vi "Adv_GetControlCurrentCapabilities.vi"(8 "error in (no error)":errorcluster, 9 "Setting":T1(ring), 10 "Control":refnum<vi>, 11 "LightField Automation in":refnum<class "LightField Automation.lvclass">) -> (0 "error out":errorcluster, 3 "LightField Automation out":refnum<class "LightField Automation.lvclass">)   [LabVIEW 2013, in "LightField Automation.lvclass"]
uses:
  LightField Automation.lvclass
  C:/Program Files/Princeton Instruments/LightField/PrincetonInstruments.LightFieldAddInSupportServices.dll
  Program Files/Princeton Instruments/LightField/PrincetonInstruments.LightFieldAddInSupportServices.dll
  LightField Automation.lvclass/LightField Automation.ctl
  C:/Program Files/Princeton Instruments/LightField/AddInViews/PrincetonInstruments.LightFieldViewV3.dll
  Program Files/Princeton Instruments/LightField/AddInViews/PrincetonInstruments.LightFieldViewV3.dll
  <vilib>/Utility/error.llb/DialogType.ctl
  TypeDefs/CalibrationLightSource.ctl
  TypeDefs/ADCGain.ctl
  TypeDefs/ADCQuality.ctl
  TypeDefs/CCDCharacteristics.ctl
  TypeDefs/CosmicRayCorrectionMethod.ctl
  TypeDefs/DateFormat.ctl
  TypeDefs/EMIccdGainControlMode.ctl
  TypeDefs/FileFormatLocation.ctl
  TypeDefs/FrameCombinationMethod.ctl
  TypeDefs/IntensifierOptions.ctl
  TypeDefs/IntensifierStatus.ctl
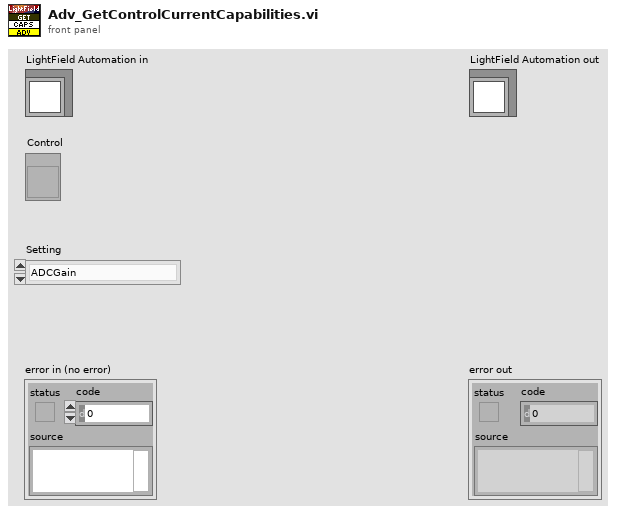
[diagram p1: front panel]
types:
  T1 = enum16{"ADCGain", "ADCQuality", "CalibrationLightSource", "CalibrationMode", "CcdCharacteristics", "CosmicRayCorrectionMethod", "DateFormat", "EMIccdGainControlMode", "FeatureProvider", "FileFormatLocation", "FrameCombinationMethod", "GateTracking", "GatingMode", "GatingSpeed", "IEMGainControlMode", "ImageOrientation", "IntensifierOptions", "IntensifierStatus", "ModulationTracking", "OpticalPortLocation", "OpticalPortShutterType", "OpticalPortType", "OutputSignal", "PhosphorType", "PhotocathodeSensitivity", "PhotonDetectionMode", "PixelDataFormat", "PixelFormat", "ReadoutControlMode", "ReadoutOrientation", "RegionsOfInterestSelection", "SensorTemperatureStatus", "SensorType", "ShutterAccessoryTimingMode", "ShutterTimingMode", "TimeFormat", "TimeStamps", "TriggerCoupling", "TriggerDetermination", "TriggerResponse", "TriggerSource", "TriggerTermination"}
  T2 = typedef "DialogType.ctl" = u16
  T3 = typedef "LVStringsAndValuesArrayTypeDef.ctl" = cluster{"String":string, "Value":ext}[]
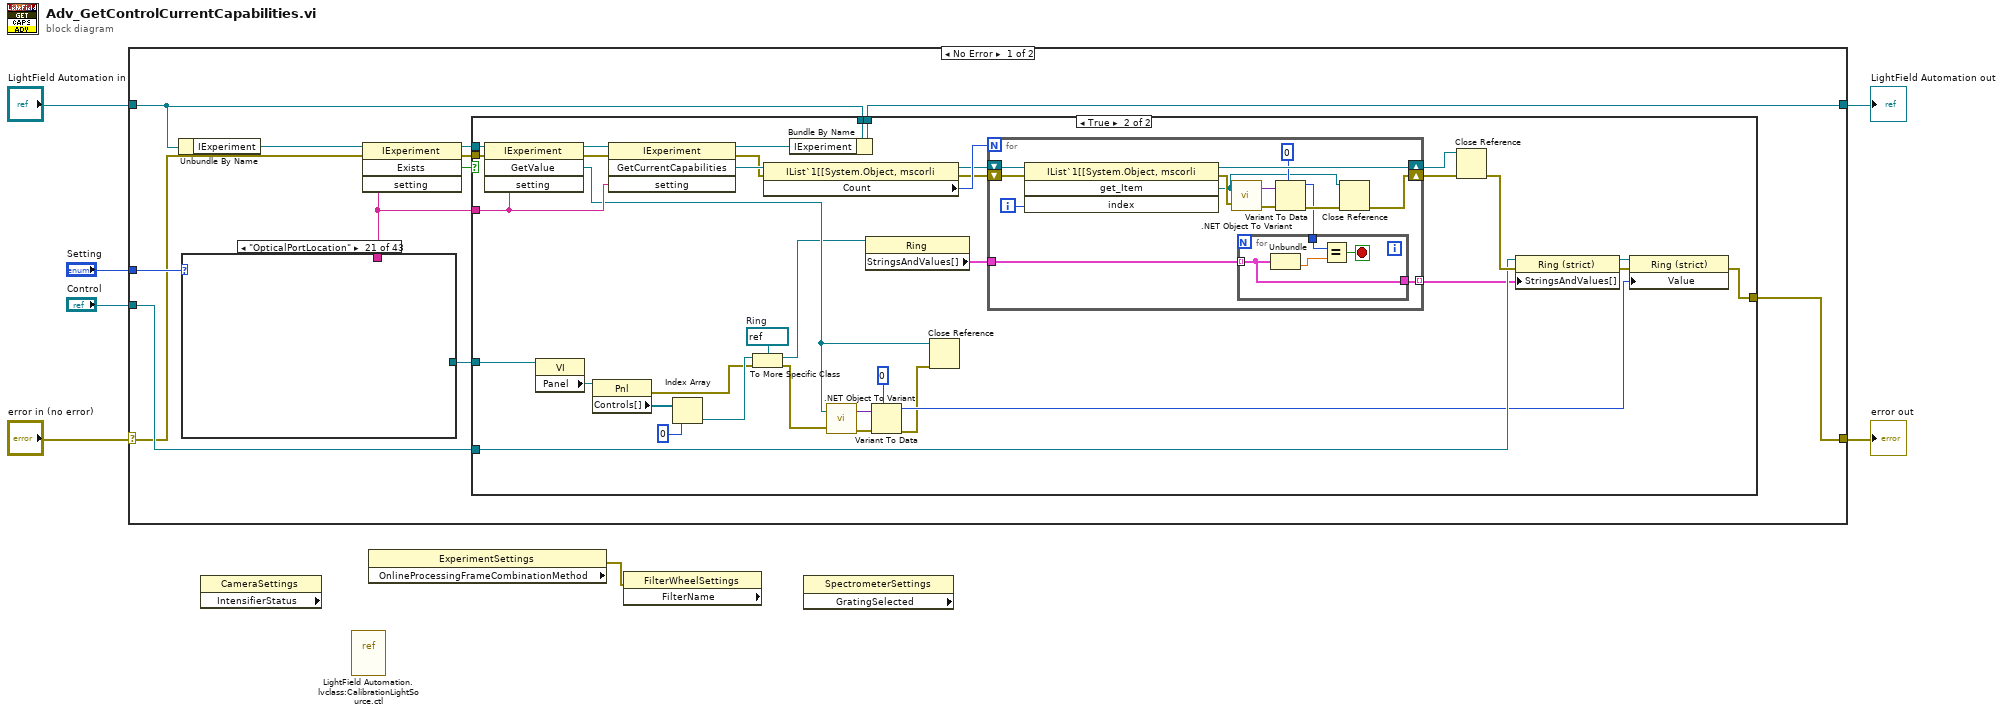
[diagram p0: block diagram]
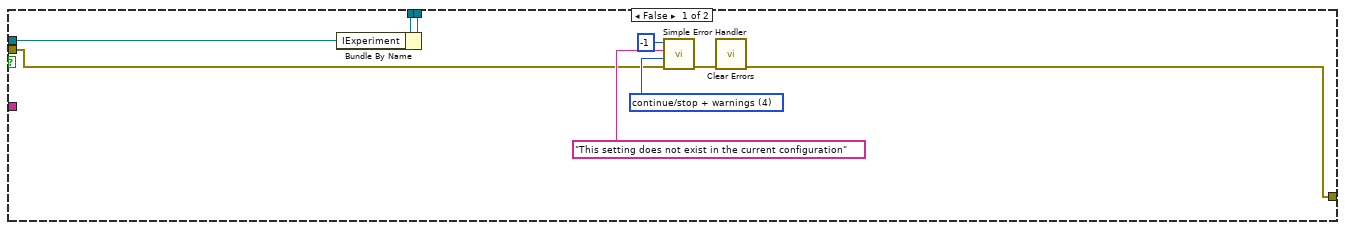
[diagram p2: hidden frame]
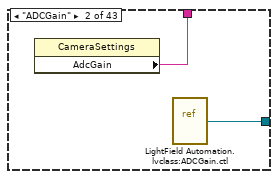
[diagram p4: hidden frame]
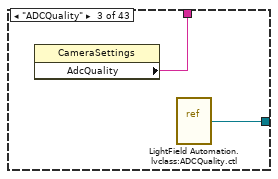
[diagram p5: hidden frame]
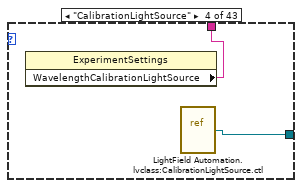
[diagram p6: hidden frame]
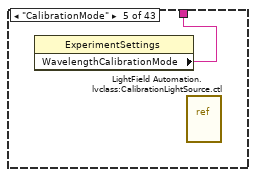
[diagram p7: hidden frame]
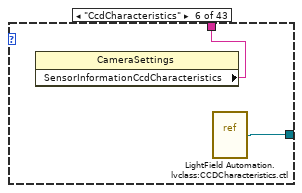
[diagram p8: hidden frame]
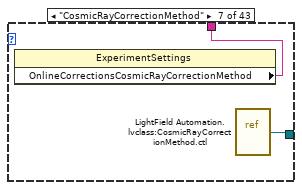
[diagram p9: hidden frame]
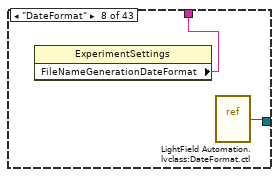
[diagram p10: hidden frame]
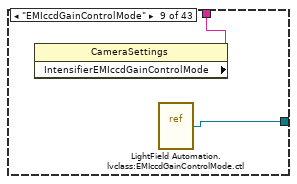
[diagram p11: hidden frame]
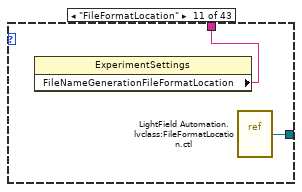
[diagram p13: hidden frame]
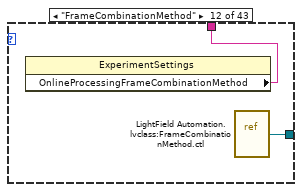
[diagram p14: hidden frame]
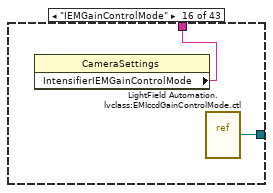
[diagram p18: hidden frame]
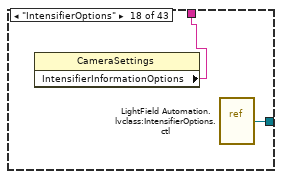
[diagram p20: hidden frame]
diagram:
  n1 = case shown="No Error" "error in (no error)" {
    selector: "error in (no error)" -> [w9 w110]
    tunnel: [w15 w110] -> w6
    tunnel: [w18 w109] -> w4
    tunnel: "LightField Automation in" -> [w19 w109]
    tunnel: "Control" -> [w17 _]
    tunnel: "Setting" -> [w16 _]
    frame No Error {
      n2 = Unbundle By Name(w19) -> ("IExperiment"=w10:refnum<k24>)
      n3 = case shown="\"OpticalPortLocation\"" w16 {
        tunnel: [_ w85 w87 w89 w90 w92 w94 w96 w98 _ w100 w102 _ _ _ w104 _ w105 w107 _ _ _ _ _ _ _ _ _ _ _ _ _ _ _ _ _ _ _ _ _ _ _ _] -> w8
        tunnel: [_ w84 w86 w88 _ w91 w93 w95 w97 _ w99 w101 _ _ _ w103 _ w106 w108 _ _ _ _ _ _ _ _ _ _ _ _ _ _ _ _ _ _ _ _ _ _ _ _] -> w14
        frame Default {
        }
        frame "ADCGain" {
          n4 = property class="CameraSettings"() -> ("AdcGain"=w85:string)  [unwired: 2 in, 2 out]
          n5 = vi-ref "LightField Automation.lvclass:ADCGain.ctl"() -> (w84:refnum<vi>)
        }
        frame "ADCQuality" {
          n6 = property class="CameraSettings"() -> ("AdcQuality"=w87:string)  [unwired: 2 in, 2 out]
          n7 = vi-ref "LightField Automation.lvclass:ADCQuality.ctl"() -> (w86:refnum<vi>)
        }
        frame "CalibrationLightSource" {
          n8 = property class="ExperimentSettings"() -> ("WavelengthCalibrationLightSource"=w89:string)  [unwired: 2 in, 2 out]
          n9 = vi-ref "LightField Automation.lvclass:CalibrationLightSource.ctl"() -> (w88:refnum<vi>)
        }
        frame "CalibrationMode" {
          n10 = property class="ExperimentSettings"() -> ("WavelengthCalibrationMode"=w90:string)  [unwired: 2 in, 2 out]
          n11 = vi-ref "LightField Automation.lvclass:CalibrationLightSource.ctl"() -> ()  [unwired: 1 out]
        }
        frame "CcdCharacteristics" {
          n12 = property class="CameraSettings"() -> ("SensorInformationCcdCharacteristics"=w92:string)  [unwired: 2 in, 2 out]
          n13 = vi-ref "LightField Automation.lvclass:CCDCharacteristics.ctl"() -> (w91:refnum<vi>)
        }
        frame "CosmicRayCorrectionMethod" {
          n14 = property class="ExperimentSettings"() -> ("OnlineCorrectionsCosmicRayCorrectionMethod"=w94:string)  [unwired: 2 in, 2 out]
          n15 = vi-ref "LightField Automation.lvclass:CosmicRayCorrectionMethod.ctl"() -> (w93:refnum<vi>)
        }
        frame "DateFormat" {
          n16 = property class="ExperimentSettings"() -> ("FileNameGenerationDateFormat"=w96:string)  [unwired: 2 in, 2 out]
          n17 = vi-ref "LightField Automation.lvclass:DateFormat.ctl"() -> (w95:refnum<vi>)
        }
        frame "EMIccdGainControlMode" {
          n18 = property class="CameraSettings"() -> ("IntensifierEMIccdGainControlMode"=w98:string)  [unwired: 2 in, 2 out]
          n19 = vi-ref "LightField Automation.lvclass:EMIccdGainControlMode.ctl"() -> (w97:refnum<vi>)
        }
        frame "FeatureProvider" {
        }
        frame "FileFormatLocation" {
          n20 = property class="ExperimentSettings"() -> ("FileNameGenerationFileFormatLocation"=w100:string)  [unwired: 2 in, 2 out]
          n21 = vi-ref "LightField Automation.lvclass:FileFormatLocation.ctl"() -> (w99:refnum<vi>)
        }
        frame "FrameCombinationMethod" {
          n22 = property class="ExperimentSettings"() -> ("OnlineProcessingFrameCombinationMethod"=w102:string)  [unwired: 2 in, 2 out]
          n23 = vi-ref "LightField Automation.lvclass:FrameCombinationMethod.ctl"() -> (w101:refnum<vi>)
        }
        frame "GateTracking" {
        }
        frame "GatingMode" {
        }
        frame "GatingSpeed" {
        }
        frame "IEMGainControlMode" {
          n24 = property class="CameraSettings"() -> ("IntensifierIEMGainControlMode"=w104:string)  [unwired: 2 in, 2 out]
          n25 = vi-ref "LightField Automation.lvclass:EMIccdGainControlMode.ctl"() -> (w103:refnum<vi>)
        }
        frame "ImageOrientation" {
        }
        frame "IntensifierOptions" {
          n26 = property class="CameraSettings"() -> ("IntensifierInformationOptions"=w105:string)  [unwired: 2 in, 2 out]
          n27 = vi-ref "LightField Automation.lvclass:IntensifierOptions.ctl"() -> (w106:refnum<vi>)
        }
        frame "IntensifierStatus" {
          n28 = property class="CameraSettings"() -> ("IntensifierStatus"=w107:string)  [unwired: 2 in, 2 out]
          n29 = vi-ref "LightField Automation.lvclass:IntensifierStatus.ctl"() -> (w108:refnum<vi>)
        }
        frame "ModulationTracking" {
        }
        frame "OpticalPortLocation" {
        }
        frame "OpticalPortShutterType" {
        }
        frame "OpticalPortType" {
        }
        frame "OutputSignal" {
        }
        frame "PhosphorType" {
        }
        frame "PhotocathodeSensitivity" {
        }
        frame "PhotonDetectionMode" {
        }
        frame "PixelDataFormat" {
        }
        frame "PixelFormat" {
        }
        frame "ReadoutControlMode" {
        }
        frame "ReadoutOrientation" {
        }
        frame "RegionsOfInterestSelection" {
        }
        frame "SensorTemperatureStatus" {
        }
        frame "SensorType" {
        }
        frame "ShutterAccessoryTimingMode" {
        }
        frame "ShutterTimingMode" {
        }
        frame "TimeFormat" {
        }
        frame "TimeStamps" {
        }
        frame "TriggerCoupling" {
        }
        frame "TriggerDetermination" {
        }
        frame "TriggerResponse" {
        }
        frame "TriggerSource" {
        }
        frame "TriggerTermination" {
        }
      }
      n30 = invoke class="IExperiment" method="Exists"(reference=w10, error in=w9, "setting"=w8) -> (reference out=w12:refnum<k24>, error out=w11:errorcluster, "Exists"=w13:bool)  [unwired: 1 in, 1 out]
      n31 = case shown="True" w13 {
        tunnel: w19 -> [w27 w65]
        tunnel: [w26 w64] -> w18
        tunnel: w17 -> [_ w57]
        tunnel: w12 -> [w28 w53]
        tunnel: w11 -> [w21 w50]
        tunnel: w8 -> [_ w46]
        tunnel: [w20 w39] -> w15
        tunnel: w14 -> [_ w31]
        frame False {
          w22 = T2 4 items=["no dialog", "OK message", "continue or stop message", "OK message + warnings", "continue/stop + warnings"] ("type of dialog (OK msg:1)")
          n32 = Bundle By Name(cluster=w27, "IExperiment"=w28) -> (w26:refnum<class "LightField Automation.lvclass">)
          n33 = call <vilib>:"Simple Error Handler.vi"("error code (no error:0)"=-1, "error source (\" \")"="This setting does not exist in the current configuration" ("source"), "type of dialog (OK msg:1)"=w22, "error in (no error)"=w21) -> ("error out"=w23:errorcluster)  [unwired: 1 in, 4 out]
          n34 = call <vilib>:"Clear Errors.vi"("error in (no error)"=w23) -> ("error out"=w20:errorcluster)  [unwired: 6 in]
        }
        frame True {
          w33 = refnum<vi> refnum  # Ring
          n35 = invoke class="IExperiment" method="GetValue"(reference=w53, error in=w50, "setting"=w46) -> (reference out=w52:refnum<k24>, error out=w51:errorcluster, "GetValue"=w41:refnum<k24>)  [unwired: 1 in, 1 out]
          n36 = property class="VI"(reference=w31) -> ("Panel"=w37:refnum<vi>)  [unwired: 1 in, 2 out]
          n37 = property class="Pnl"(reference=w37) -> (error out=w30:errorcluster, "Controls[]"=w36:refnum<vi>[])  [unwired: 1 in, 1 out]
          n38 = invoke class="IExperiment" method="GetCurrentCapabilities"(reference=w52, error in=w51, "setting"=w46) -> (reference out=w56:refnum<k24>, error out=w54:errorcluster, "GetCurrentCapabilities"=w55:refnum<k24>)  [unwired: 1 in, 1 out]
          n39 = Index Array(array=w36, index=0) -> (element=w34:refnum<vi>)
          n40 = To More Specific Class(target class=w33, reference=w34, error in=w30) -> (specific class reference=w32:refnum<vi>, error out=w29:errorcluster)
          n41 = property class="IList`1[[System.Object, mscorli"(reference=w55, error in=w54) -> (reference out=w62:refnum<k24>, error out=w61:errorcluster, "Count"=w63:i32)
          n42 = Bundle By Name(cluster=w65, "IExperiment"=w56) -> (w64:refnum<class "LightField Automation.lvclass">)
          n43 = call <vilib>:".NET Object To Variant.vi"("error in (no error)"=w29, ".NET object"=w41) -> ("error out"=w49:errorcluster, "variant"=w48:variant)
          n44 = property class="Ring"(reference=w32) -> ("StringsAndValues[]"=w38:T3)  [unwired: 1 in, 2 out]
          n45 = Variant To Data(error in=w49, type=0, Variant=w48) -> (data=w43:i32, error out=w42:errorcluster)
          n46 = Close Reference(reference=w41, error in (no error)=w42) -> ()  [unwired: 1 out]
          n47 = for {
            N: w63 -> [_]
            shift-right: [w76] -> w59
            shift-left: w62 -> [w79]
            shift-right: [w70] -> w60
            shift-left: w61 -> [w78]
            tunnel: w38 -> [w68]
            tunnel: [w66] -> w40 mode=indexing
            i -> [w77]
            n48 = invoke class="IList`1[[System.Object, mscorli" method="get_Item"(reference=w79, error in=w78, "index"=w77) -> (reference out=w76:refnum<k24>, error out=w73:errorcluster, "get_Item"=w69:refnum<k24>)  [unwired: 1 in, 1 out]
            n49 = call <vilib>:".NET Object To Variant.vi"("error in (no error)"=w73, ".NET object"=w69) -> ("error out"=w75:errorcluster, "variant"=w74:variant)
            n50 = Variant To Data(error in=w75, type=0, Variant=w74) -> (data=w67:i32, error out=w71:errorcluster)
            n51 = for {
              tunnel: w68 -> [w80] mode=indexing
              tunnel: w67 -> [w83]
              tunnel: [w80] -> w66
              stop <- w81 stop-if-true
              n52 = Unbundle(w80) -> ("Value"=w82:ext)  [unwired: 1 out]
              n53 = Equal?(x=w83, y=w82) -> (x = y?=w81:bool)
            }
            n54 = Close Reference(reference=w69, error in (no error)=w71) -> (error out=w70:errorcluster)
          }
          n55 = Close Reference(reference=w59, error in (no error)=w60) -> (error out=w58:errorcluster)
          n56 = property class="Ring (strict)"(reference=w57, error in=w58, "StringsAndValues[]"=w40) -> (reference out=w45:refnum<vi>, error out=w44:errorcluster)
          n57 = property class="Ring (strict)"(reference=w45, error in=w44, "Value"=w43) -> (error out=w39:errorcluster)  [unwired: 1 out]
        }
      }
    }
    frame Error {
    }
  }
  "error out" <- w6
  "LightField Automation out" <- w4
  n58 = property class="CameraSettings" props=["IntensifierStatus"]() -> ()  [unwired: 2 in, 3 out]
  n59 = vi-ref "LightField Automation.lvclass:CalibrationLightSource.ctl"() -> ()  [unwired: 1 out]
  n60 = property class="ExperimentSettings" props=["OnlineProcessingFrameCombinationMethod"]() -> (error out=w1:errorcluster)  [unwired: 2 in, 2 out]
  n61 = property class="FilterWheelSettings" props=["FilterName"](error in=w1) -> ()  [unwired: 1 in, 3 out]
  n62 = property class="SpectrometerSettings" props=["GratingSelected"]() -> ()  [unwired: 2 in, 3 out]
